vi "GateControllerTest.vi"() -> ()   [LabVIEW 2021]
panel:
  out "read buffer":string
  in  "VISA resource name":refnum<visa-resource-name>="COM6"
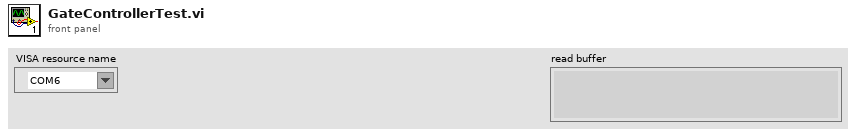
[diagram p1: front panel]
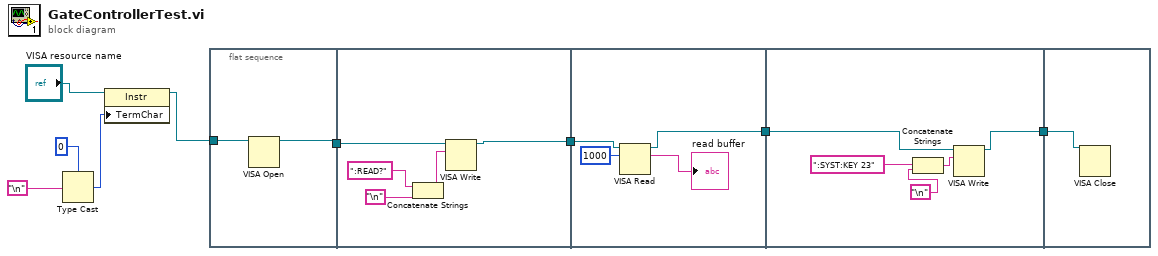
[diagram p0: block diagram]
diagram:
  n1 = Type Cast(type=i8 0, x="\n") -> (*(type *) &x=w1:i8)
  n2 = property class="Instr"(reference="VISA resource name", "TermChar"=w1) -> (reference out=w4:refnum<visa-resource-name>)  [unwired: 1 in, 1 out]
  n3 = flat-sequence {
    tunnel: [w11] -> w9
    tunnel: w4 -> [w10]
    tunnel: w9 -> [w16]
    tunnel: [w15] -> w8
    tunnel: w8 -> [w19]
    tunnel: [w18] -> w7
    tunnel: w7 -> [w25]
    tunnel: [w24] -> w6
    tunnel: w6 -> [w26]
    frame #0 {
      n4 = VISA Open(VISA resource name=w10) -> (VISA resource name=w11:refnum<visa-resource-name>)  [unwired: 4 in, 1 out]
    }
    frame #1 {
      n5 = Concatenate Strings(":READ?" ("write buffer"), "\n") -> (w12:string)
      n6 = VISA Write(VISA resource name=w16, write buffer=w12) -> (VISA resource name out=w15:refnum<visa-resource-name>)  [unwired: 1 in, 2 out]
    }
    frame #2 {
      n7 = VISA Read(VISA resource name=w19, byte count=u32 1000) -> (VISA resource name out=w18:refnum<visa-resource-name>, read buffer=→"read buffer":string)  [unwired: 1 in, 2 out]
    }
    frame #3 {
      n8 = Concatenate Strings(":SYST:KEY 23", "\n") -> (w22:string)
      n9 = VISA Write(VISA resource name=w25, write buffer=w22) -> (VISA resource name out=w24:refnum<visa-resource-name>)  [unwired: 1 in, 2 out]
    }
    frame #4 {
      n10 = VISA Close(VISA resource name=w26) -> ()  [unwired: 1 in, 1 out]
    }
  }
